vi "Create-log-file.vi"(8 "error in (no error)":errorcluster, 11 "Errors in":T1) -> (0 "error out":errorcluster, 3 "Errors out":T1)   [LabVIEW 2013, in "CameraVision.lvlib" / "CV-Errors.lvclass"]
uses:
  CV-Errors.lvclass
  Object-reference.ctl
  CV-Errors.lvclass/CV-Errors.ctl
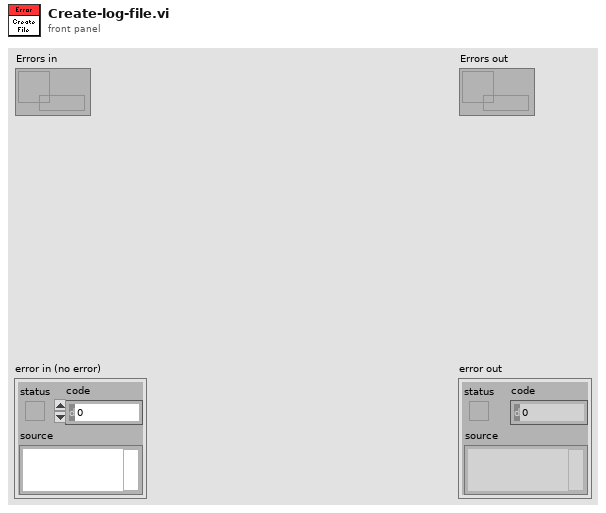
[diagram p1: front panel]
types:
  T1 = typedef "CameraVision.lvlib/CV-Errors.lvclass/Object-reference.ctl" = refnum<data-value>
  T2 = enum16{"open", "replace", "create", "open or create", "replace or create", "replace or create with confirmation"}
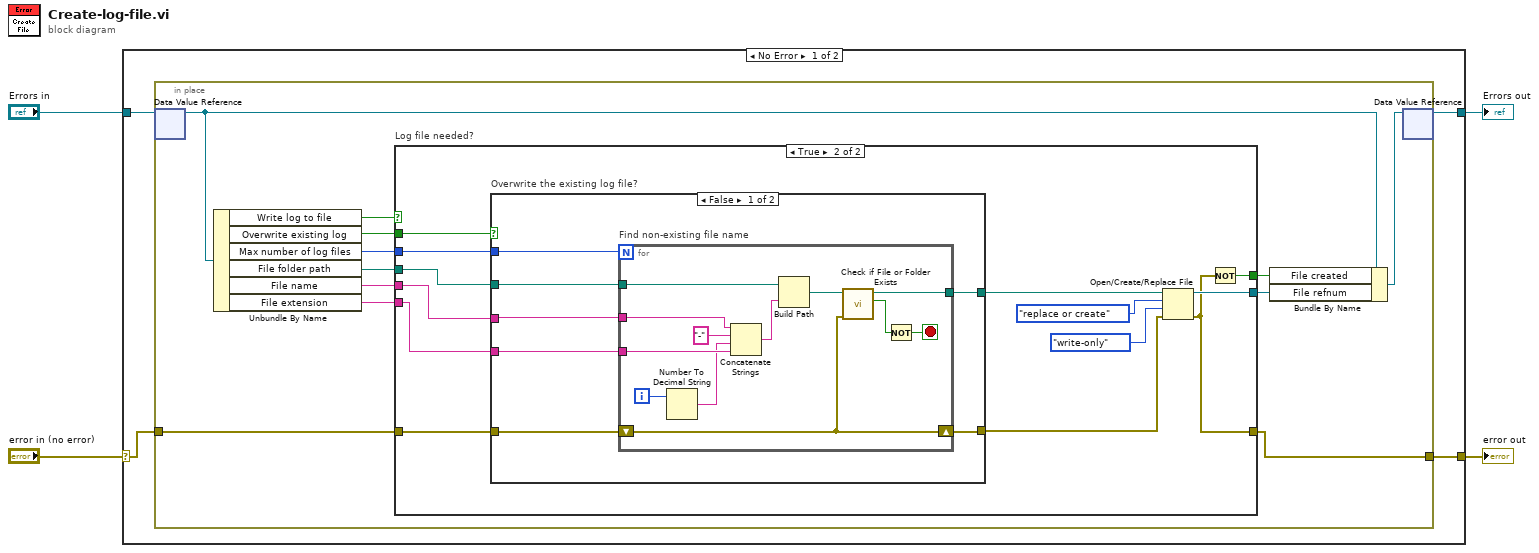
[diagram p0: block diagram]
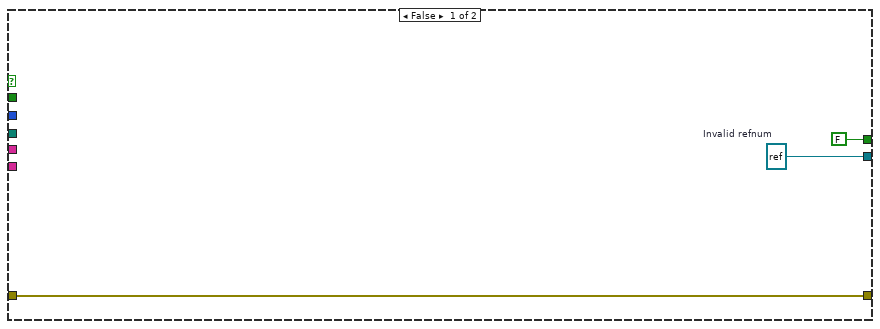
[diagram p2: hidden frame]
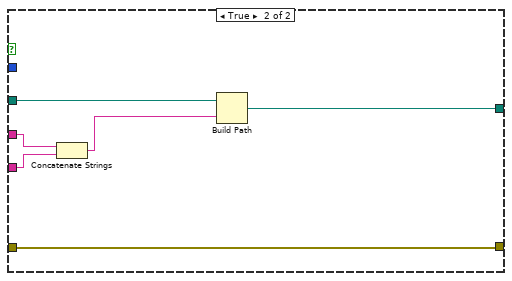
[diagram p3: hidden frame]
diagram:
  n1 = case shown="No Error" "error in (no error)" {
    selector: "error in (no error)" -> [w8 w63]
    tunnel: [w7 w63] -> w3
    tunnel: [w5 w62] -> w1
    tunnel: "Errors in" -> [w6 w62]
    frame No Error {
      n2 = in-place {
        in-place-border: w8 -> [w13]
        in-place-border: [w12] -> w7
        n3 = in-place-dvr #1(w6) -> (w10:refnum<class "CV-Errors.lvclass">)  [unwired: 1 out]
        n4 = Unbundle By Name(w10) -> ("Write log to file"=w20:bool, "Overwrite existing log"=w18:bool, "Max number of log files"=w11:i32, "File folder path"=w19:path, "File name"=w17:string, "File extension"=w16:string)
        n5 = case "Log file needed?" shown="True" w20 {
          tunnel: w19 -> [_ w24]
          tunnel: w18 -> [_ w36]
          tunnel: w13 -> [w23 w35]
          tunnel: [w23 w28] -> w12
          tunnel: [w22 w30] -> w14
          tunnel: [FALSE w29] -> w15
          tunnel: w17 -> [_ w27]
          tunnel: w16 -> [_ w26]
          tunnel: w11 -> [_ w25]
          frame False {
            w22 = refnum<file> refnum  # Invalid refnum
          }
          frame True {
            n6 = case "Overwrite the existing log file?" shown="False" w36 {
              tunnel: [w40 w60] -> w32
              tunnel: w24 -> [w43 w61]
              tunnel: w35 -> [w42 w59]
              tunnel: [w41 w59] -> w31
              tunnel: w27 -> [w39 w58]
              tunnel: w26 -> [w38 w57]
              tunnel: w25 -> [w37 _]
              frame False {
                n7 = for "Find non-existing file name" {
                  N: w37 -> [_]
                  tunnel: w43 -> [w55]
                  tunnel: w38 -> [w51]
                  tunnel: w39 -> [w52]
                  tunnel: [w49] -> w40
                  shift-right: [w44] -> w41
                  shift-left: w42 -> [w44]
                  i -> [w54]
                  stop <- w47 stop-if-true
                  n8 = Number To Decimal String(number=w54) -> (decimal integer string=w46:string)  [unwired: 1 in]
                  n9 = Concatenate Strings(w52, "-" ("string"), w46, w51) -> (w53:string)
                  n10 = Build Path(base path=w55, name or relative path=w53) -> (appended path=w50:path)
                  n11 = call <vilib>:"Check if File or Folder Exists.vi"("error in (no error)"=w44, "path"=w50) -> ("file or folder exists?"=w48:bool, "dup path"=w49:path)  [unwired: 7 in, 1 out]
                  n12 = Not(x=w48) -> (.not. x?=w47:bool)
                }
              }
              frame True {
                n13 = Concatenate Strings(w58, w57) -> (w56:string)
                n14 = Build Path(base path=w61, name or relative path=w56) -> (appended path=w60:path)
              }
            }
            n15 = Open/Create/Replace File(file path (use dialog)=w32, error in=w31, operation (0:open)=T2."replace or create", access (0:read/write)=enum16{"read/write", "read-only", "write-only"}."write-only") -> (refnum out=w30:refnum<file>, error out=w28:errorcluster)  [unwired: 2 in, 1 out]
            n16 = Not(x=w28) -> (.not. x?=w29:bool)
          }
        }
        n17 = Bundle By Name(cluster=w10, "File created"=w15, "File refnum"=w14) -> (w9:refnum<class "CV-Errors.lvclass">)
        n18 = in-place-dvr #1(w9) -> (w5:T1)  [unwired: 1 out]
      }
    }
    frame Error {
    }
  }
  "error out" <- w3
  "Errors out" <- w1
